vi "Reserve Registered Sessions.vi"(6 "timeout (ms)":i32=10000, 8 "error in":errorcluster, 9 "instrument type id":string) -> (0 "error out":errorcluster, 3 "session reservation out":refnum<class "Session Reservation.lvclass">)   [LabVIEW 2020, in "NI Session Management V1 Client.lvlib" / "Session Reservation.lvclass"]
doc: "Reserves all registered session(s) with the specified <b>instrument type id</b>. If the <b>instrument type id</b> is an empty string, reserves all registered sessions for all instrument types."
uses:
  Session Reservation.lvclass
  gRPC/Generated APIs/ni/measurementlink/sessionmanagement/v1/RPC Messages/ni_measurementlink_sessionmanagement_v1_ReserveAllRegisteredSessionsRequest.ctl
  gRPC/Generated APIs/ni/measurementlink/sessionmanagement/v1/RPC Messages/ni_measurementlink_PinMapContext.ctl
  IReservation Observer/IReservation Observer.lvclass
  gRPC/Generated APIs/ni/measurementlink/sessionmanagement/v1/RPC Messages/ni_measurementlink_sessionmanagement_v1_ReserveSessionsResponse.ctl
  gRPC/Generated APIs/ni/measurementlink/sessionmanagement/v1/RPC Messages/ni_measurementlink_sessionmanagement_v1_SessionInformation.ctl
  gRPC/Generated APIs/ni/measurementlink/sessionmanagement/v1/RPC Messages/nidevice_grpc_Session.ctl
  gRPC/Generated APIs/ni/measurementlink/sessionmanagement/v1/RPC Messages/ni_measurementlink_sessionmanagement_v1_ChannelMapping.ctl
  gRPC/Generated APIs/ni/measurementlink/sessionmanagement/v1/RPC Messages/ni_measurementlink_sessionmanagement_v1_MultiplexerSessionInformation.ctl
  gRPC/Generated APIs/ni/measurementlink/sessionmanagement/v1/RPC Messages/ni_measurementlink_sessionmanagement_v1_ReserveSessionsResponse_GroupMappingsEntry.ctl
  gRPC/Generated APIs/ni/measurementlink/sessionmanagement/v1/RPC Messages/ni_measurementlink_sessionmanagement_v1_ResolvedPinsOrRelays.ctl
  gRPC/Generated APIs/ni/measurementlink/sessionmanagement/v1/ni.measurementlink.sessionmanagement.v1.api.lvlib
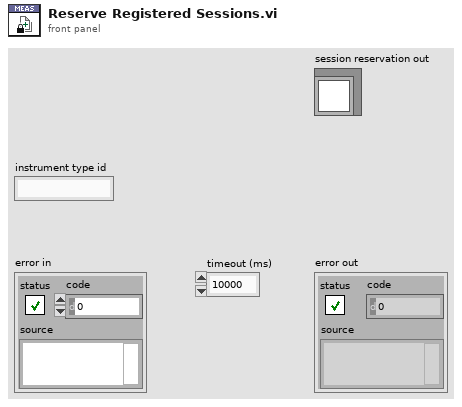
[diagram p1: front panel]
types:
  T1 = typedef "ni.measurementlink.sessionmanagement.v1.api.lvlib/ni_measurementlink_sessionmanagement_v1_ReserveSessionsResponse.ctl" = cluster{"sessions":T2[], "multiplexer_sessions":T5[], "group_mappings":T6[]}
  T2 = typedef "ni.measurementlink.sessionmanagement.v1.api.lvlib/ni_measurementlink_sessionmanagement_v1_SessionInformation.ctl" = cluster{"session":T3, "resource_name":string, "channel_list":string, "instrument_type_id":string, "session_exists":bool, "channel_mappings":T4[]}
  T3 = typedef "ni.measurementlink.sessionmanagement.v1.api.lvlib/nidevice_grpc_Session.ctl" = cluster{"name":string}
  T4 = typedef "ni.measurementlink.sessionmanagement.v1.api.lvlib/ni_measurementlink_sessionmanagement_v1_ChannelMapping.ctl" = cluster{"pin_or_relay_name":string, "site":i32, "channel":string, "multiplexer_resource_name":string, "multiplexer_route":string}
  T5 = typedef "ni.measurementlink.sessionmanagement.v1.api.lvlib/ni_measurementlink_sessionmanagement_v1_MultiplexerSessionInformation.ctl" = cluster{"session":T3, "resource_name":string, "multiplexer_type_id":string, "session_exists":bool}
  T6 = typedef "ni.measurementlink.sessionmanagement.v1.api.lvlib/ni_measurementlink_sessionmanagement_v1_ReserveSessionsResponse_GroupMappingsEntry.ctl" = cluster{"key":string, "value":T7}
  T7 = typedef "ni.measurementlink.sessionmanagement.v1.api.lvlib/ni_measurementlink_sessionmanagement_v1_ResolvedPinsOrRelays.ctl" = cluster{"pin_or_relay_names":string[]}
  T8 = typedef "ni.measurementlink.sessionmanagement.v1.api.lvlib/ni_measurementlink_PinMapContext.ctl" = cluster{"pin_map_id":string, "sites":i32[]}
  T9 = typedef "ni.measurementlink.sessionmanagement.v1.api.lvlib/ni_measurementlink_sessionmanagement_v1_ReserveAllRegisteredSessionsRequest.ctl" = cluster{"timeout_in_milliseconds":i32, "instrument_type_id":string}
  T10 = typedef "ni.measurementlink.sessionmanagement.v1.api.lvlib/ni_measurementlink_sessionmanagement_v1_ReserveAllRegisteredSessionsResponse.ctl" = cluster{"sessions":T2[]}
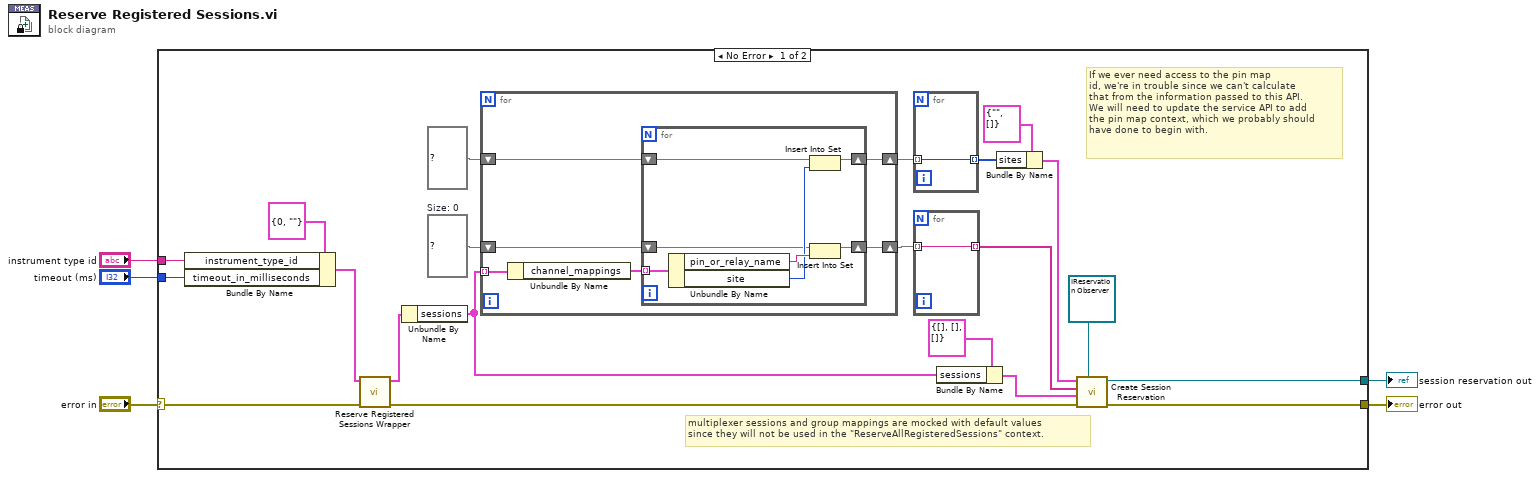
[diagram p0: block diagram]
diagram:
  n1 = case shown="No Error" "error in" {
    selector: "error in" -> [w25 w42]
    tunnel: "instrument type id" -> [w24 _]
    tunnel: "timeout (ms)" -> [w23 _]
    tunnel: [w21 _] -> w3
    tunnel: [w19 w42] -> w4
    frame No Error {
      w16 = set{string} {}  # Size: 0
      # "multiplexer sessions and group mappings are mocked with default values\nsince they will not be used in the \"ReserveAllRegisteredSessions\" context."
      # "If we ever need access to the pin map\nid, we're in trouble since we can't calculate\nthat from the information passed to this API.\nWe will need to update the service API to add\nthe pin map context, which we probably should\nhave done to begin with."
      n2 = Bundle By Name(cluster=T9 {"timeout_in_milliseconds"=0, "instrument_type_id"=""} ("Request Data"), "instrument_type_id"=w24, "timeout_in_milliseconds"=w23) -> (w22:T9)
      n3 = call "Reserve Registered Sessions Wrapper.vi"("error in"=w25, "request data"=w22) -> ("error out"=w20:errorcluster, "response data"=w18:T10)  [unwired: 8 in]
      n4 = Unbundle By Name(w18) -> ("sessions"=w6:T2[])
      n5 = for {
        tunnel: w6 -> [w34] mode=indexing
        shift-right: [w30] -> w15
        shift-left: w16 -> [w29]
        shift-right: [w31] -> w14
        shift-left: set{i32} {} ("set in") -> [w32]
        n6 = Unbundle By Name(w34) -> ("channel_mappings"=w33:T4[])
        n7 = for {
          tunnel: w33 -> [w41] mode=indexing
          shift-right: [w36] -> w30
          shift-left: w29 -> [w35]
          shift-right: [w37] -> w31
          shift-left: w32 -> [w38]
          n8 = Unbundle By Name(w41) -> ("pin_or_relay_name"=w40:string, "site"=w39:i32)
          n9 = Insert Into Set(10:w39, 11:w38) -> (3:w37:set{i32})  [unwired: 1 out]
          n10 = Insert Into Set(10:w40, 11:w35) -> (3:w36:set{string})  [unwired: 1 out]
        }
      }
      n11 = for {
        tunnel: [w27] -> w11 mode=indexing
        tunnel: w14 -> [w27] mode=indexing
      }
      n12 = for {
        tunnel: [w28] -> w13 mode=indexing
        tunnel: w15 -> [w28] mode=indexing
      }
      n13 = Bundle By Name(cluster=T1 {"sessions"=[], "multiplexer_sessions"=[], "group_mappings"=[]} ("session reservation response"), "sessions"=w6) -> (w7:T1)
      n14 = Bundle By Name(cluster=T8 {"pin_map_id"="", "sites"=[]} ("pin map context"), "sites"=w11) -> (w10:T8)
      n15 = call "Create Session Reservation.vi"("reservation observer"=refnum<class "IReservation Observer.lvclass"> refnum, "error in"=w20, "session reservation response"=w7, "pin or relay names"=w13, "pin map context"=w10) -> ("error out"=w19:errorcluster, "session reservation out"=w21:refnum<class "Session Reservation.lvclass">)  [unwired: 5 in]
    }
    frame Error {
    }
  }
  "error out" <- w4
  "session reservation out" <- w3
